vi "Insert Conditional Branch.vi"(6 "Insertion Index":i32=-1, 7 "Parent ID":string, 8 "error in (no error)":errorcluster, 9 "Unique ID":string, 10 "Name":string, 11 "Test Executive in":refnum<class "Test Executive.lvclass">) -> (0 "error out":errorcluster, 1 "Replaced?":bool, 3 "Test Executive out":refnum<class "Test Executive.lvclass">, 5 "Unique ID out":string)   [LabVIEW 2017, in "Test Executive.lvlib" / "Test Executive.lvclass"]
uses:
  <vilib>/gpm_packages/@cs/test-executive/Source/Test Executive/TestExecutive/Test Executive.lvclass
  <vilib>/gpm_packages/@cs/test-executive/Source/Test Executive/Conditional Branch/Conditional Branch.lvclass
  <vilib>/gpm_packages/@cs/test-executive/Source/Test Executive/TestExecutive/Test Executive.lvclass/Test Executive.ctl
  86c3a7d6-a696-4c16-aacc-1d76e87cd5a8.vi
  <vilib>/gpm_packages/@cs/linked-list/Source/Linked List/ILinkedList/ILinked List.lvclass
  <vilib>/gpm_packages/@cs/linked-list/Source/Linked List/Linked List Ref/Linked List Ref.lvclass
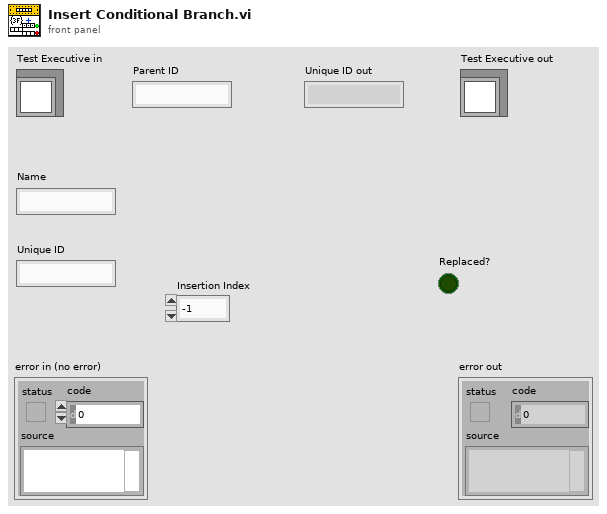
[diagram p1: front panel]
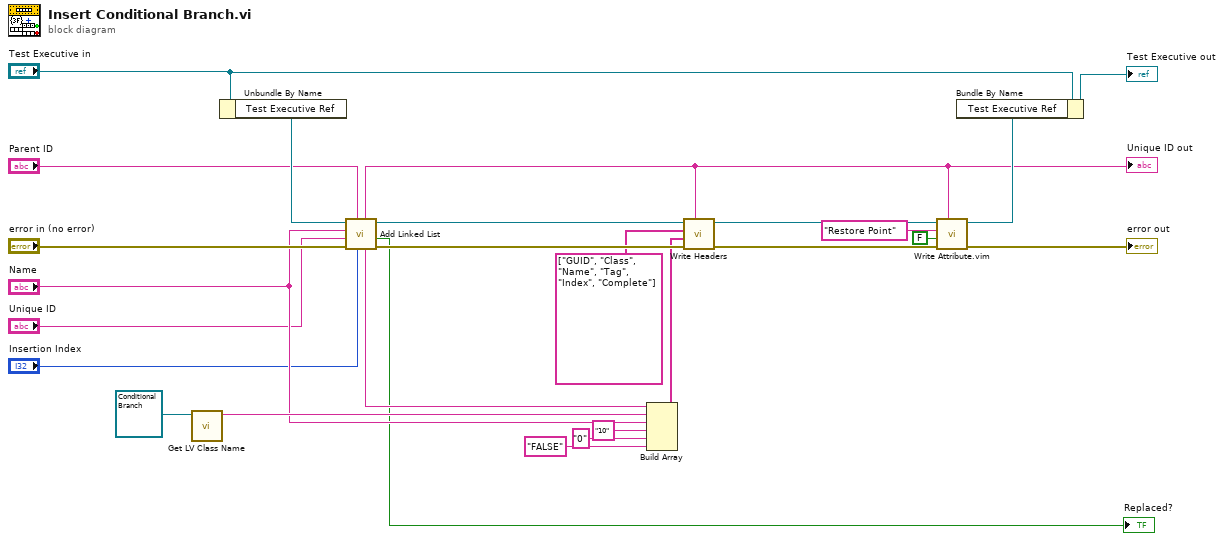
[diagram p0: block diagram]
diagram:
  n1 = call <vilib>:"Get LV Class Name.vi"("object"=refnum<class "Conditional Branch.lvclass"> refnum ("Test Executive.lvlib:Conditional Branch.lvclass")) -> ("class name"=w21:string)  [unwired: 9 in, 1 out]
  n2 = Unbundle By Name("Test Executive in") -> ("Test Executive Ref"=w25:refnum<data-value>)
  n3 = call <vilib>:"Add Linked List.vi"("Insertion Index"="Insertion Index", "Parent ID"="Parent ID", "error in (no error)"="error in (no error)", "Linked List ID"="Unique ID", "Name"="Name", "Linked List Ref"=w25) -> ("error out"=w23:errorcluster, "Replaced?"=→"Replaced?":bool, "Linked List Ref out"=w24:refnum<data-value>, "Linked List ID out"=w10:string)  [unwired: 2 in]
  "Unique ID out" <- w10
  n4 = Build Array(w10, w21, "Name", "10" ("element"), "0" ("element"), "FALSE" ("element")) -> (w19:string[])
  n5 = call <vilib>:"Write Headers.vi"("Linked List ID"=w10, "error in (no error)"=w23, "Header Values"=w19, "Header Names"=string[] ["GUID", "Class", "Name", "Tag", "Index", "Complete"], "Linked List Ref"=w24) -> ("error out"=w15:errorcluster, "Linked List Ref out"=w16:refnum<data-value>)  [unwired: 5 in]
  n6 = call "Write Attribute.vim"("Linked List ID"=w10, "error in (no error)"=w15, "Attribute"=FALSE, "Attribute Name"="Restore Point", "Linked List Ref"=w16) -> ("error out"=→"error out":errorcluster, "Linked List Ref out"=w14:refnum<data-value>)  [unwired: 3 in, 2 out]
  n7 = Bundle By Name(cluster="Test Executive in", "Test Executive Ref"=w14) -> (→"Test Executive out":refnum<class "Test Executive.lvclass">)
